vi "Launcher.vi"() -> ()   [LabVIEW 2017]
uses:
  Controls/Coordinates.ctl
panel:
  in  "Exit":bool
  in  "Option":bool
  in  "Start":bool
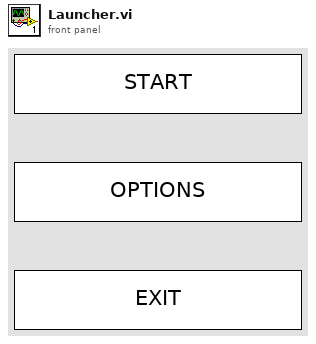
[diagram p1: front panel]
types:
  T1 = typedef "Coordinates.ctl" = cluster{"X":i32, "Y":i32}
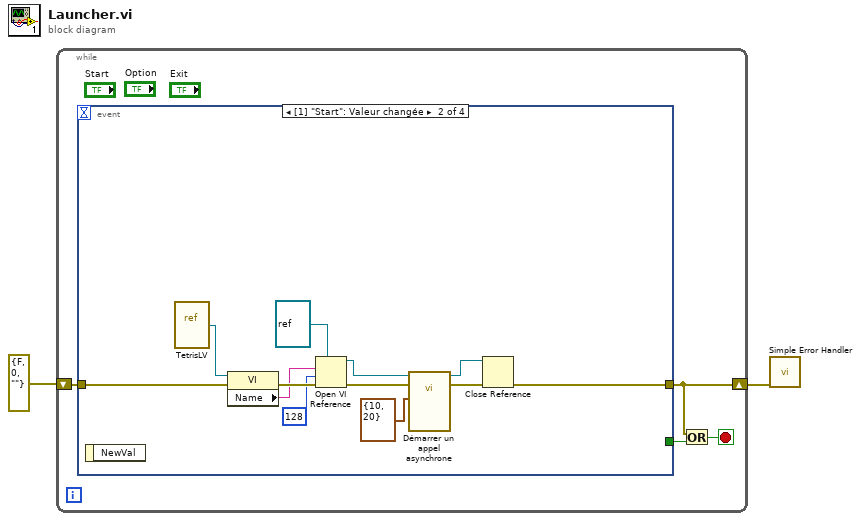
[diagram p0: block diagram]
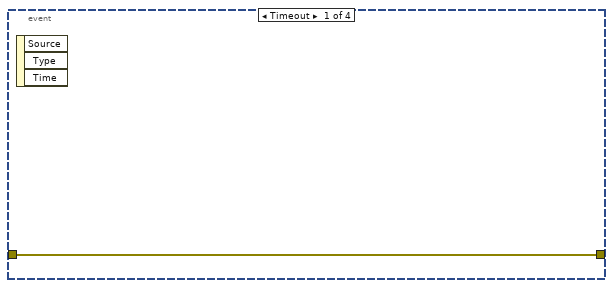
[diagram p2: hidden frame]
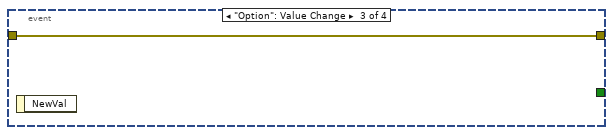
[diagram p3: hidden frame]
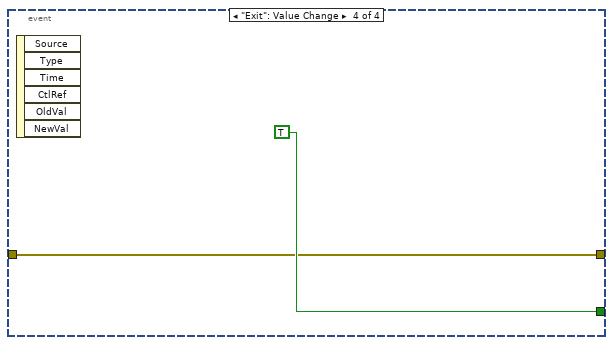
[diagram p4: hidden frame]
diagram:
  n1 = while {
    shift-right: [w3] -> w1
    shift-left: errorcluster {"status"=FALSE, "code"=0, "source"=""} ("constante d'erreur") -> [w5]
    stop <- w4 stop-if-true
    n2 = event shown="[1] \"Start\": Valeur changée" {
      selector: _ -> [_ _ _ _]
      dyn-events: _ -> [_ _ _ _]
      timeout: _ -> [_ _ _ _]
      tunnel: [_ _ _ TRUE] -> w6
      tunnel: w5 -> [w7 w19 w20 w21]
      tunnel: [w7 w12 w20 w21] -> w3
      event Timeout {
        n3 = event-data() -> ()  [unwired: 1 in, 3 out]
      }
      event "Start": Value Change {
        n4 = event-data() -> ()  [unwired: 1 in, 1 out]
        n5 = vi-ref "TetrisLV.vi"() -> (w16:refnum<vi>)
        n6 = property class="VI"(reference=w16, error in=w19) -> (error out=w18:errorcluster, "Name"=w17:string)  [unwired: 1 out]
        n7 = Open VI Reference(type specifier VI Refnum (for type only)=refnum<vi> refnum ("spécificateur de type du refnum de VI (pour type seulement)"), vi path=w17, options=128, error in (no error)=w18) -> (vi reference=w8:refnum<vi>, error out=w9:errorcluster)  [unwired: 2 in]
        n8 = call-by-ref "Démarrer un appel asynchrone"(reference=w8, error in=w9, "Board Size"=T1 {"X"=10, "Y"=20}) -> (reference out=w13:refnum<vi>, error out=w14:errorcluster)  [unwired: 11 in]
        n9 = Close Reference(reference=w13, error in (no error)=w14) -> (error out=w12:errorcluster)
      }
      event "Option": Value Change {
        n10 = event-data() -> ()  [unwired: 1 in, 1 out]
      }
      event "Exit": Value Change {
        n11 = event-data() -> ()  [unwired: 1 in, 6 out]
      }
    }
    n12 = Or(x=w3, y=w6) -> (x .or. y?=w4:bool)
  }
  n13 = call <vilib>:"Simple Error Handler.vi"("error in (no error)"=w1) -> ()  [unwired: 4 in, 5 out]
